vi "corridor_edge_check.vi"(1 "min tack length":dbl, 2 "corridor width":dbl, 3 "Waypoint X Coordinate":dbl, 4 "angle":dbl) -> (0 "Out of Corridor":bool)   [LabVIEW 2013]
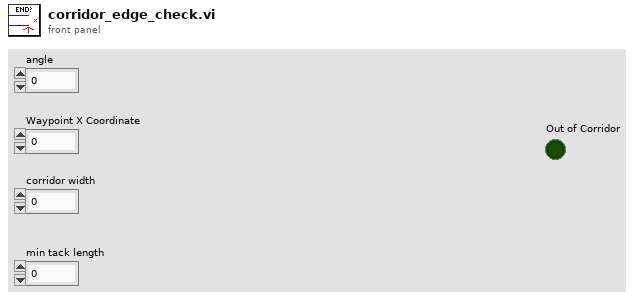
[diagram p1: front panel]
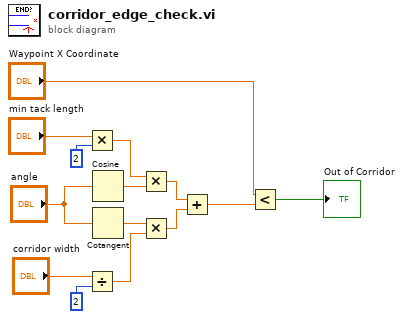
[diagram p0: block diagram]
diagram:
  n1 = Multiply(x="min tack length", y=2) -> (x*y=w8:dbl)
  n2 = Divide(x="corridor width", y=2) -> (x/y=w6:dbl)
  n3 = Cosine(x="angle") -> (cos(x)=w9:dbl)
  n4 = Cotangent(1:"angle") -> (0:w7:dbl)
  n5 = Multiply(x=w8, y=w9) -> (x*y=w5:dbl)
  n6 = Multiply(x=w7, y=w6) -> (x*y=w4:dbl)
  n7 = Add(x=w5, y=w4) -> (x+y=w2:dbl)
  n8 = Less?(x="Waypoint X Coordinate", y=w2) -> (x < y?=→"Out of Corridor":bool)
